vi "Caudal.vi"() -> ()   [LabVIEW 2021]
uses:
  <vilib>/NI/Modbus Library/API/Modbus API.lvclass/Modbus API.ctl
  <vilib>/NI/Modbus Library/Transmission Data Unit/Transmission Data Unit.lvclass/Transmission Data Unit.ctl
  <vilib>/NI/Modbus Library/Transmission Data Unit/Write Unit ID.vi
  <vilib>/NI/Modbus Library/API/Read Transmission Data Unit.vi
  <vilib>/NI/Modbus Library/API/Write Transmission Data Unit.vi
  <vilib>/NI/Modbus Library/API/Master/Modbus Master.lvclass
  C:/Program Files (x86)/National Instruments/LabVIEW 2021/vi.lib/NI/Modbus Library/API/Modbus API.lvclass
  <vilib>/NI/Modbus Library/API/Wrapper/Create TCP Master.vi
  <vilib>/NI/Modbus Library/API/Wrapper/API Main.lvlib
panel:
  in  "Tab Control":enum32{"Scada", "Config"}(tab)
  out "Caudal":dbl
  out "Consumo":dbl
  out "Gauge":dbl(knob) scale=0.0..30.0
  in  "Precio del agua":dbl=1.0
  out "Total":dbl format="Q.%#_6g"
  in  "address":string="192.168.50.147"
  in  "Puerto":u16=502
  in  "ID":u8=1
  # "Consumo de Agua"
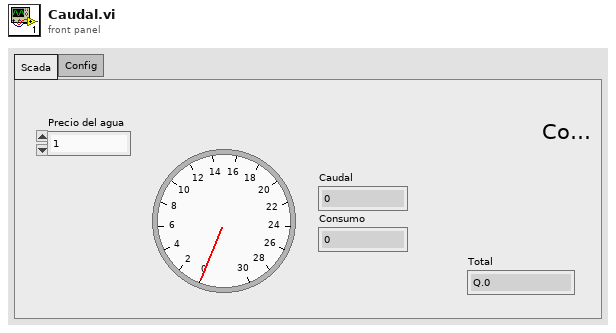
[diagram p1: front panel]
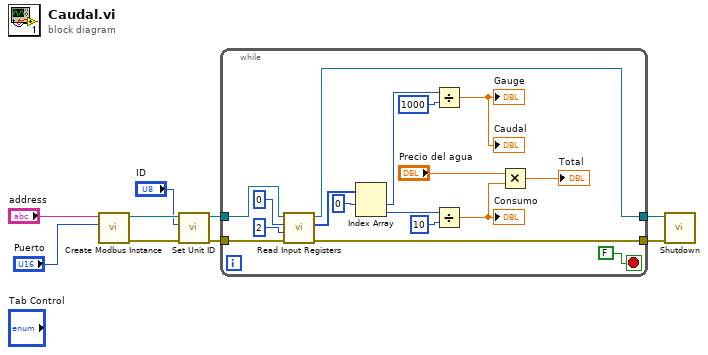
[diagram p0: block diagram]
diagram:
  n1 = call-poly <vilib>:"Create Modbus Instance.vi"("port (502)"="Puerto", "address"="address") -> ("error out"=w8:errorcluster, "TCP master instance"=w9:refnum<class "Modbus Master.lvclass">)  [unwired: 8 in]
  n2 = call <vilib>:"Set Unit ID.vi"("error in"=w8, "unit ID"="ID", "Modbus master in"=w9) -> ("error out"=w3:errorcluster, "Modbus master out"=w4:refnum<class "Modbus Master.lvclass">)  [unwired: 7 in]
  n3 = while {
    tunnel: w3 -> [w25]
    tunnel: [w21] -> w1
    tunnel: w4 -> [w26]
    tunnel: [w22] -> w2
    stop <- FALSE stop-if-true
    n4 = call-dynamic "Read Input Registers.vi"("error in"=w25, "number of inputs"=u16 2, "starting address"=u16 0, "Modbus master in"=w26) -> ("error out"=w21:errorcluster, "register values"=w19:u16[], "Modbus master out"=w22:refnum<class "Modbus Master.lvclass">)  [unwired: 5 in]
    n5 = Index Array(array=w19, index #1=0 ("index")) -> (element #1=w17:u16, element #2=w14:u16)  [unwired: 1 in]
    n6 = Divide(x=w17, y=u16 1000) -> (x/y=→"Caudal" →"Gauge":dbl)
    n7 = Divide(x=w14, y=u16 10) -> (x/y=w11:dbl)
    "Consumo" <- w11
    n8 = Multiply(x="Precio del agua", y=w11) -> (x*y=→"Total":dbl)
  }
  n9 = call-dynamic "Shutdown.vi"("error in"=w1, "Modbus master in"=w2) -> ()  [unwired: 9 in, 1 out]
